vi "Dead Zone.vi"(1 "Dead Value":dbl, 2 "Data":dbl, 3 "Range":dbl) -> (0 "Dead Zoned Data":dbl)   [LabVIEW 2014]
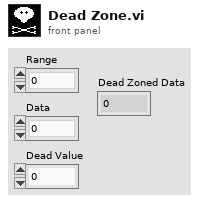
[diagram p1: front panel]
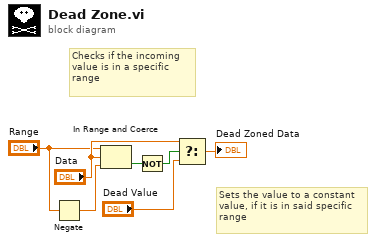
[diagram p0: block diagram]
diagram:
  # "Sets the value to a constant value, if it is in said specific range"
  # "Checks if the incoming value is in a specific range"
  n1 = Negate(x="Range") -> (-x=w7:dbl)
  n2 = In Range and Coerce(upper limit="Range", x="Data", lower limit=w7) -> (In Range?=w6:bool)  [unwired: 1 out]
  n3 = Not(x=w6) -> (.not. x?=w5:bool)
  n4 = Select(t="Data", s=w5, f="Dead Value") -> (s? t:f=→"Dead Zoned Data":dbl)
